vi "Read Timestamp Configuration.vi"(8 "error in (no error)":errorcluster, 9 "Default If Not Found":timestamp, 10 "Name":string, 11 "IniFileSection in":refnum<class "IniFileSection.lvclass">) -> (0 "error out":errorcluster, 1 "Not Found?":bool, 2 "Value":timestamp, 3 "IniFileSection out":refnum<class "IniFileSection.lvclass">)   [LabVIEW 2020, in "IniFileSection.lvclass"]
uses:
  <vilib>/gpm_packages/@cs/Configuration/Source/IniFileSection/IniFileSection.lvclass
  <vilib>/gpm_packages/@cs/Configuration/Source/IniFileSection/IniFileSection.lvclass/IniFileSection.ctl
  <vilib>/Utility/config.llb/Read Key (String).vi
  <vilib>/Utility/config.llb/NI_LVConfig.lvlib
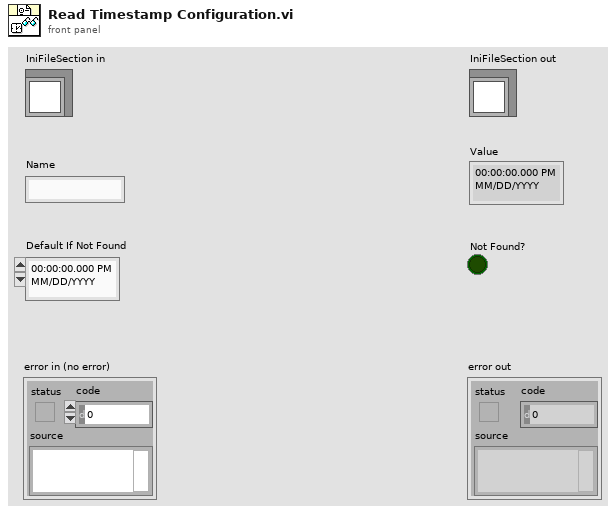
[diagram p1: front panel]
types:
  T1 = typedef "NI_LVConfig.lvlib/Config Data RefNum.ctl" = refnum<k1>
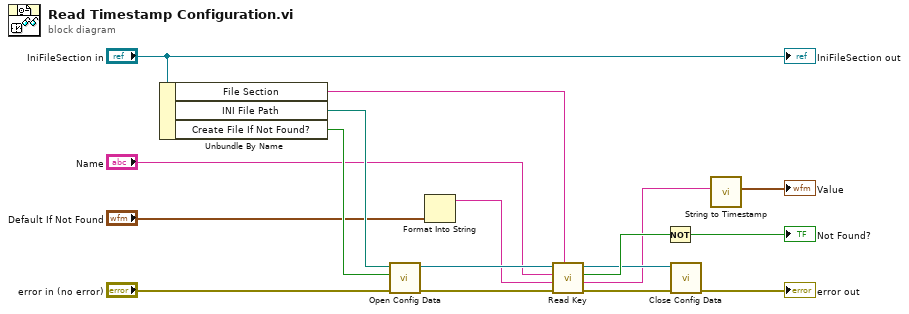
[diagram p0: block diagram]
diagram:
  n1 = Unbundle By Name("IniFileSection in") -> ("File Section"=w6:string, "INI File Path"=w13:path, "Create File If Not Found?"=w12:bool)
  n2 = call <vilib>:"Open Config Data.vi"("error in (no error)"="error in (no error)", "create file if necessary (T)"=w12, "configuration file path"=w13) -> ("error out"=w10:errorcluster, "refnum"=w17:T1)  [unwired: 6 in, 1 out]
  n3 = Format Into String("Default If Not Found") -> (resulting string=w2:string)  [unwired: 3 in, 1 out]
  n4 = call-poly <vilib>:"Read Key.vi"("section"=w6, "error in (no error)"=w10, "default value"=w2, "key"="Name", "refnum"=w17) -> ("error out"=w9:errorcluster, "value"=w1:string, "found?"=w11:bool, "refnum out"=w8:T1)  [unwired: 3 in]
  n5 = Not(x=w11) -> (.not. x?=→"Not Found?":bool)
  n6 = call <vilib>:"Close Config Data.vi"("error in (no error)"=w9, "refnum"=w8) -> ("error out"=→"error out":errorcluster)  [unwired: 8 in, 1 out]
  n7 = call <vilib>:"String to Timestamp.vi"("Timestamp String"=w1) -> ("Timestamp"=→"Value":timestamp)  [unwired: 10 in]
  "IniFileSection out" <- "IniFileSection in"
